vi "mtlb simx Get Object Group Data.vi"(0 "clientIDandObjectTypeAndDataTypeAndOperationMode":i32, 1 "handlesCountAndIntDataCountAndFloatDataCountAndStringDataCount":i32, 2 "handles":i32, 3 "intData":i32, 4 "floatData":sgl, 5 "stringData":string, 7 "error in (no error)":errorcluster) -> (20 "clientIDandObjectTypeAndDataTypeAndOperationMode out":i32, 21 "handlesCountAndIntDataCountAndFloatDataCountAndStringDataCount out":i32, 22 "handles out":i32, 23 "intData out":i32, 24 "floatData out":sgl, 25 "stringData out":string, 26 "function return":i32, 27 "error out":errorcluster)   [LabVIEW 2019, in "PXL_V-REP.lvlib"]
doc: "EXTAPI_DLLEXPORT simxInt mtlb_simxGetObjectGroupData(simxInt* clientIDandObjectTypeAndDataTypeAndOperationMode,simxInt* handlesCountAndIntDataCountAndFloatDataCountAndStringDataCount,simxInt** handles,simxInt** intData,simxFloat** floatData,simxChar** stringData);"
uses:
  PXL_V-REP.lvlib
  <userlib>/V-REP/remoteApi.dll
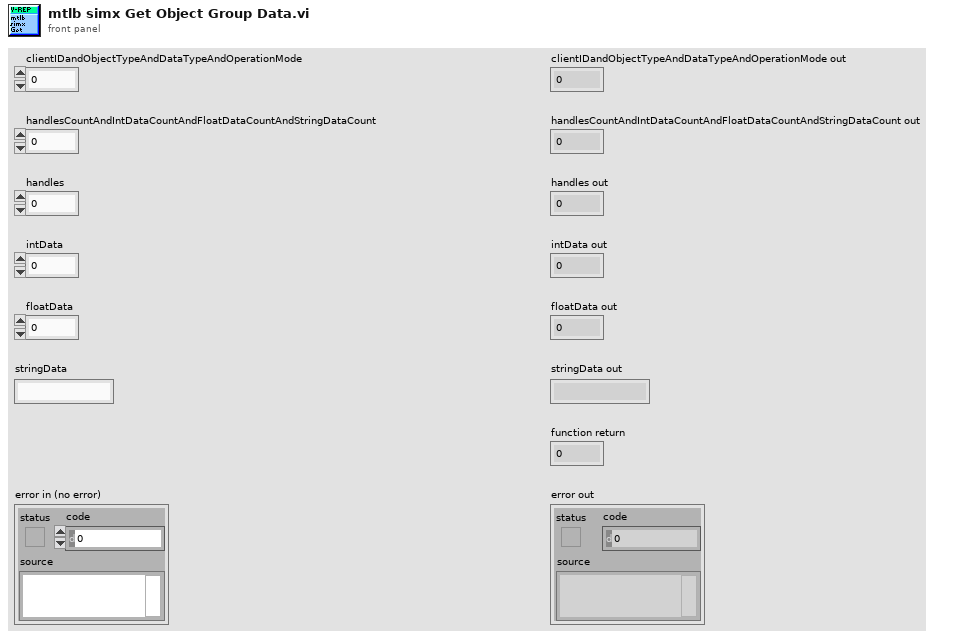
[diagram p1: front panel]
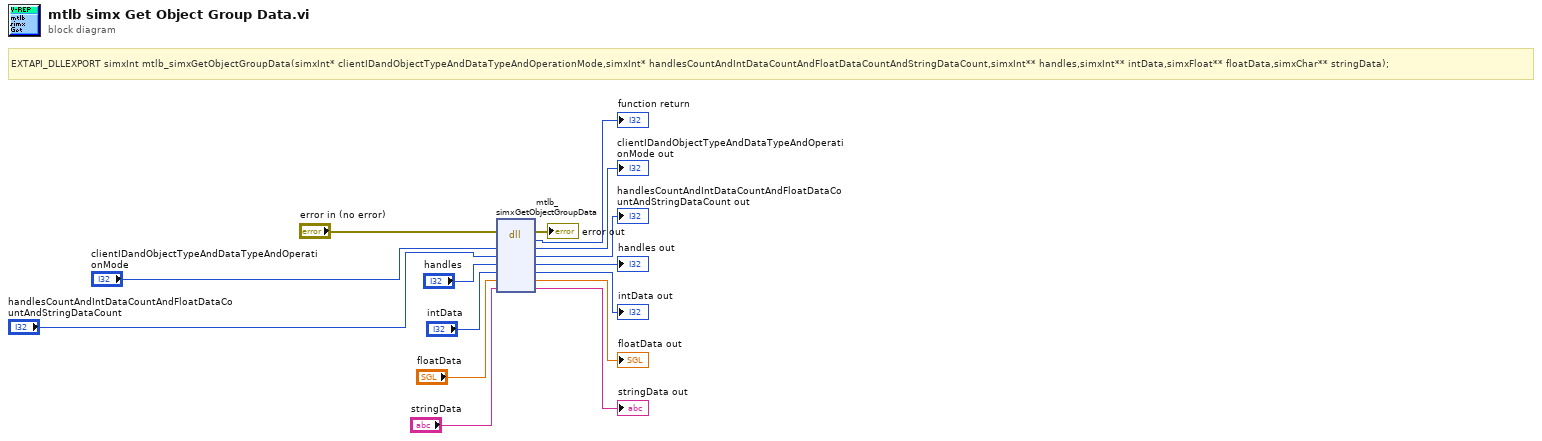
[diagram p0: block diagram]
diagram:
  # "EXTAPI_DLLEXPORT simxInt mtlb_simxGetObjectGroupData(simxInt* clientIDandObjectTypeAndDataTypeAndOperationMode,simxInt* handlesCountAndIntDataCountAndFloatDataCountAndStringDataCount,simxInt** handles,simxInt** intData,simxFloat** floatData,simxChar** stringData);"
  n1 = dll-call lib="C:/Program Files (x86)/National Instruments/LabVIEW 2019/user.lib/V-REP/remoteApi.*" fn="mtlb_simxGetObjectGroupData"(error in="error in (no error)", "clientIDandObjectTypeAndDataTypeAndOperationMode"="clientIDandObjectTypeAndDataTypeAndOperationMode", "handlesCountAndIntDataCountAndFloatDataCountAndStringDataCount"="handlesCountAndIntDataCountAndFloatDataCountAndStringDataCount", "handles"="handles", "intData"="intData", "floatData"="floatData", "stringData"="stringData") -> (error out=→"error out":errorcluster, →"function return":i32, "clientIDandObjectTypeAndDataTypeAndOperationMode"=→"clientIDandObjectTypeAndDataTypeAndOperationMode out":i32, "handlesCountAndIntDataCountAndFloatDataCountAndStringDataCount"=→"handlesCountAndIntDataCountAndFloatDataCountAndStringDataCount out":i32, "handles"=→"handles out":i32, "intData"=→"intData out":i32, "floatData"=→"floatData out":sgl, "stringData"=→"stringData out":string)  [unwired: 2 in, 1 out]
